vi "Write_RamsetePath_to_Command_List.vi"(0 "LastCmdNumb":i32=64, 4 "CmdNumb":i32=62, 5 "WayPoints":T2[](array[typedef])=[{"x"=15.0, "y"=105.0, "angle"=0.0}, {"x"=35.0, "y"=105.0, "angle"=0.0}, {"x"=210.0, "y"=32.0, "angle"=0.0}, {"x"=230.0, "y"=32.0, "angle"=0.0}], 6 "FirstCmdNumb":i32=60, 7 "Include Step":bool=TRUE, 8 "Path Sample Array":T1[](array[typedef]), 9 "Comment":string, 10 "starting step":i32, 11 "Cmd List File":path) -> ()   [LabVIEW 2019]
uses:
  Pathfinder-Lib/VIs/Waypoint.ctl
  Pathfinder-Lib/Pathfinder.lvlib
  PathExecution_Library/PATH_SAMPLE.ctl
  PathExecution_Library/PathExecution_Library.lvlib
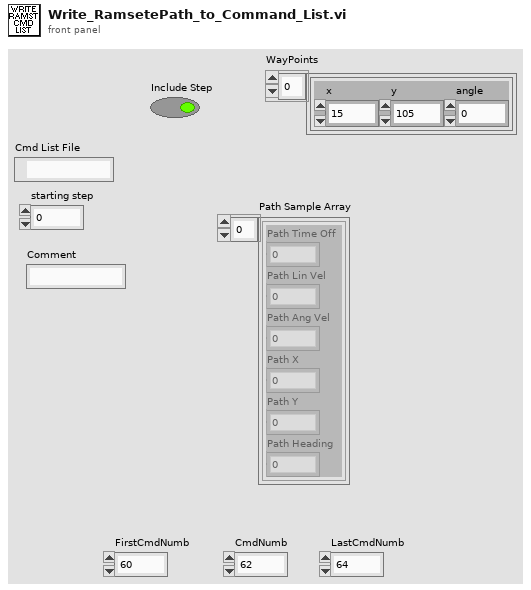
[diagram p1: front panel]
types:
  T1 = typedef "PathExecution_Library.lvlib/PATH_SAMPLE.ctl" = cluster{"Path Lin Vel":dbl, "Path Ang Vel":dbl, "Path X":dbl, "Path Y":dbl, "Path Heading":dbl, "Path Time Off":dbl}
  T2 = typedef "Pathfinder.lvlib/Waypoint.ctl" = cluster{"x":dbl, "y":dbl, "angle":dbl}
  T3 = enum16{"open", "replace", "create", "open or create", "replace or create", "replace or create with confirmation"}
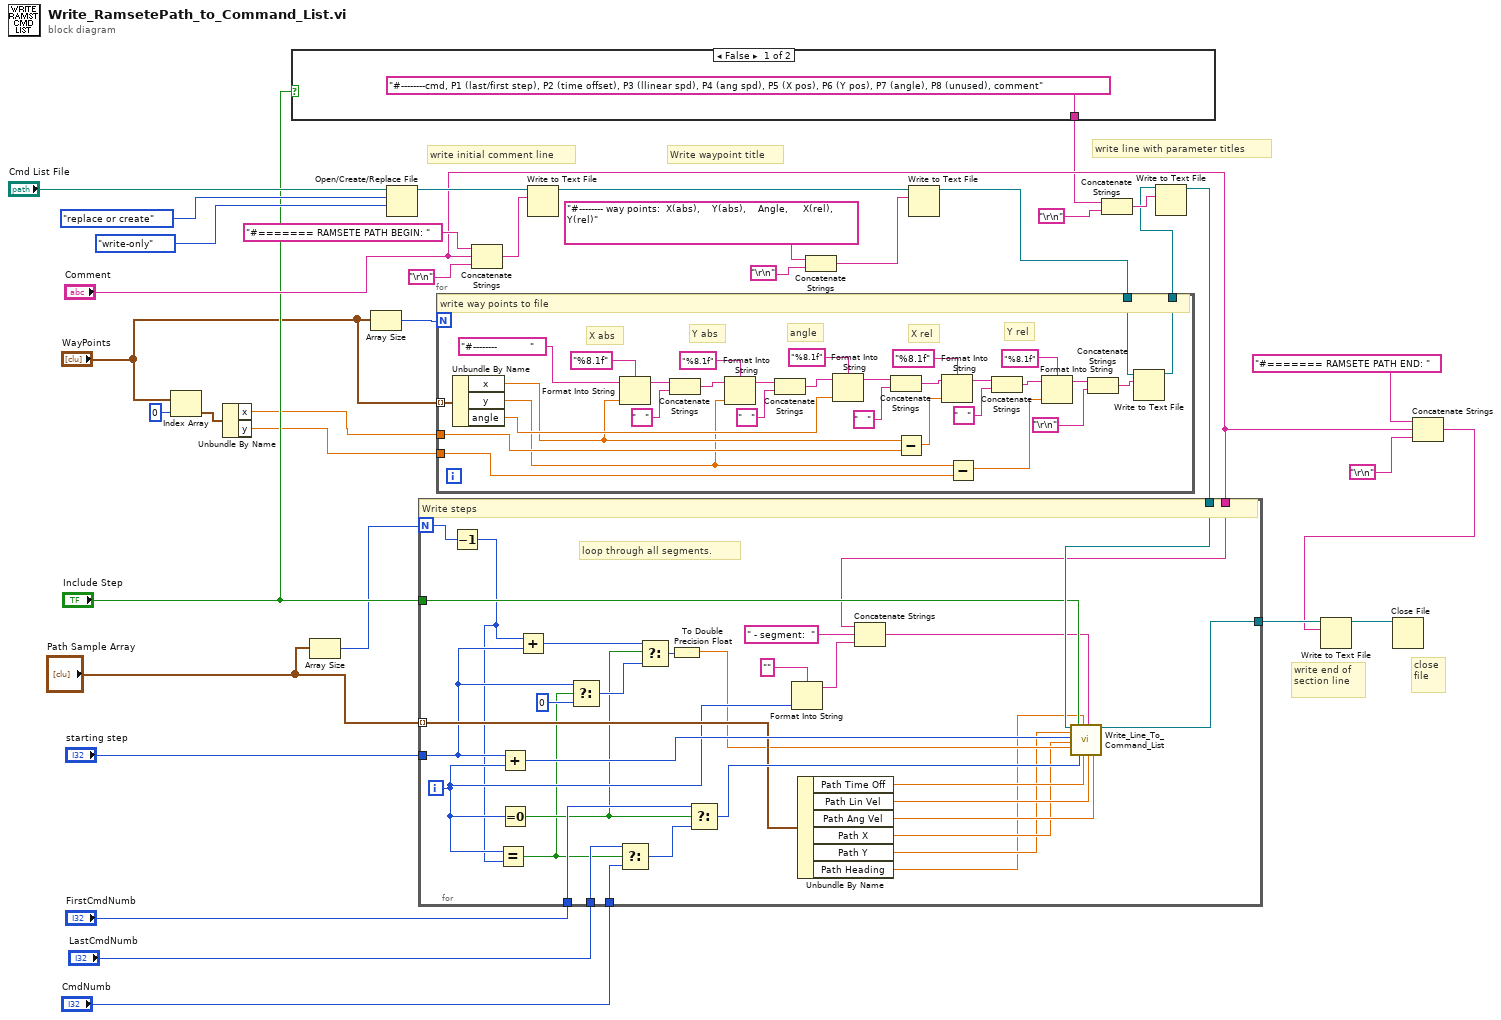
[diagram p0: block diagram]
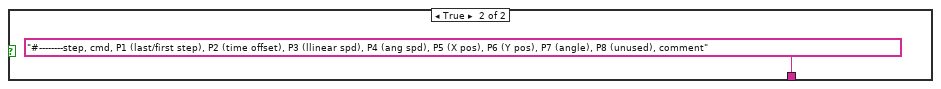
[diagram p2: hidden frame]
diagram:
  # "Write waypoint title"
  # "close\nfile"
  # "write end of\nsection line"
  # "write line with parameter titles"
  # "write initial comment line"
  n1 = Index Array(array="WayPoints", index=0) -> (element=w13:T2)
  n2 = Unbundle By Name(w13) -> ("x"=w8:dbl, "y"=w7:dbl)
  n3 = case shown="False" "Include Step" {
    tunnel: ["#--------cmd, P1 (last/first step), P2 (time offset), P3 (llinear spd), P4 (ang spd), P5 (X pos), P6 (Y pos), P7 (angle), P8 (unused), comment" ("string") "#--------step, cmd, P1 (last/first step), P2 (time offset), P3 (llinear spd), P4 (ang spd), P5 (X pos), P6 (Y pos), P7 (angle), P8 (unused), comment" ("string")] -> w16
    frame False {
    }
    frame True {
    }
  }
  n4 = Array Size(array="Path Sample Array") -> (size(s)=w1:i32)
  n5 = Array Size(array="WayPoints") -> (size(s)=w12:i32)
  n6 = Open/Create/Replace File(file path (use dialog)="Cmd List File", operation (0:open)=T3."replace or create", access (0:read/write)=enum16{"read/write", "read-only", "write-only"}."write-only") -> (refnum out=w32:refnum<file>)  [unwired: 3 in, 2 out]
  n7 = Concatenate Strings("#======= RAMSETE PATH BEGIN: " ("string"), "Comment", "\r\n") -> (w29:string)
  n8 = Write to Text File(file (use dialog)=w32, text=w29) -> (refnum out=w10:refnum<file>)  [unwired: 2 in, 2 out]
  n9 = Concatenate Strings("#-------- way points:  X(abs),    Y(abs),    Angle,     X(rel),    Y(rel)" ("string"), "\r\n") -> (w5:string)
  n10 = Write to Text File(file (use dialog)=w10, text=w5) -> (refnum out=w4:refnum<file>)  [unwired: 2 in, 2 out]
  n11 = for {
    N: w12 -> [_]
    tunnel: "WayPoints" -> [w59] mode=indexing
    tunnel: w8 -> [w58]
    tunnel: w7 -> [w57]
    tunnel: w4 -> [w54]
    tunnel: [w53] -> w3
    # "Y rel"
    # "X rel"
    # "angle"
    # "Y abs"
    # "X abs"
    # "write way points to file"
    n12 = Unbundle By Name(w59) -> ("x"=w42:dbl, "y"=w41:dbl, "angle"=w56:dbl)
    n13 = Format Into String(format string="%8.1f", initial string="#--------           " ("string"), w42) -> (resulting string=w69:string)  [unwired: 1 in, 1 out]
    n14 = Concatenate Strings(w69, "   " ("string")) -> (w67:string)
    n15 = Format Into String(format string="%8.1f", initial string=w67, w41) -> (resulting string=w68:string)  [unwired: 1 in, 1 out]
    n16 = Concatenate Strings(w68, "   " ("string")) -> (w66:string)
    n17 = Format Into String(format string="%8.1f", initial string=w66, w56) -> (resulting string=w55:string)  [unwired: 1 in, 1 out]
    n18 = Concatenate Strings(w55, "   " ("string")) -> (w49:string)
    n19 = Subtract(x=w42, y=w58) -> (x-y=w40:dbl)
    n20 = Format Into String(format string="%8.1f", initial string=w49, w40) -> (resulting string=w52:string)  [unwired: 1 in, 1 out]
    n21 = Subtract(x=w41, y=w57) -> (x-y=w39:dbl)
    n22 = Concatenate Strings(w52, "   " ("string")) -> (w48:string)
    n23 = Format Into String(format string="%8.1f", initial string=w48, w39) -> (resulting string=w44:string)  [unwired: 1 in, 1 out]
    n24 = Concatenate Strings(w44, "\r\n") -> (w43:string)
    n25 = Write to Text File(file (use dialog)=w54, text=w43) -> (refnum out=w53:refnum<file>)  [unwired: 2 in, 2 out]
  }
  n26 = Concatenate Strings(w16, "\r\n") -> (w28:string)
  n27 = Write to Text File(file (use dialog)=w3, text=w28) -> (refnum out=w31:refnum<file>)  [unwired: 2 in, 2 out]
  n28 = for {
    N: w1 -> [w95]
    tunnel: "Path Sample Array" -> [w98] mode=indexing
    tunnel: "starting step" -> [w83]
    tunnel: [w97] -> w20
    tunnel: w31 -> [w96]
    tunnel: "CmdNumb" -> [w94]
    tunnel: "LastCmdNumb" -> [w93]
    tunnel: "FirstCmdNumb" -> [w92]
    tunnel: "Include Step" -> [w91]
    tunnel: "Comment" -> [w86]
    i -> [w87]
    # "loop through all segments."
    # "Write steps"
    n29 = Decrement(x=w95) -> (x-1=w82:i32)
    n30 = Equal?(x=w87, y=w82) -> (x = y?=w76:bool)
    n31 = Add(x=w83, y=w87) -> (x+y=w101:i32)
    n32 = Equal To 0?(x=w87) -> (x = 0?=w77:bool)
    n33 = Add(x=w82, y=w83) -> (x+y=w81:i32)
    n34 = Select(t=w83, s=w76, f=0) -> (s? t:f=w84:i32)
    n35 = Select(t=w93, s=w76, f=w94) -> (s? t:f=w100:i32)
    n36 = Select(t=w81, s=w77, f=w84) -> (s? t:f=w79:i32)
    n37 = To Double Precision Float(number=w79) -> (double precision float=w78:dbl)
    n38 = Select(t=w92, s=w77, f=w100) -> (s? t:f=w99:i32)
    n39 = Format Into String(format string="", w87) -> (resulting string=w89:string)  [unwired: 2 in, 1 out]
    n40 = Unbundle By Name(w98) -> ("Path Time Off"=w75:dbl, "Path Lin Vel"=w74:dbl, "Path Ang Vel"=w73:dbl, "Path X"=w72:dbl, "Path Y"=w71:dbl, "Path Heading"=w70:dbl)
    n41 = Concatenate Strings(w86, " - segment:  " ("string"), w89) -> (w85:string)
    n42 = call "Write_Line_To_Command_List.vi"("Byte Stream File in"=w96, "P6"=w71, "Step"=w101, "P5"=w72, "P1"=w78, "Include Step"=w91, "CmdNumb"=w99, "P7"=w70, "P2"=w75, "Comment"=w85, "P3"=w74, "P4"=w73) -> ("Byte Stream File out"=w97:refnum<file>)  [unwired: 7 in]
  }
  n43 = Concatenate Strings("#======= RAMSETE PATH END: " ("string"), "Comment", "\r\n") -> (w18:string)
  n44 = Write to Text File(file (use dialog)=w20, text=w18) -> (refnum out=w19:refnum<file>)  [unwired: 2 in, 2 out]
  n45 = Close File(refnum=w19) -> ()  [unwired: 1 in, 2 out]
